vi "Initialize DAQ Channel.vi"(8 "error in (no error)":errorcluster, 10 "DAQmx Analog Channel":tag, 11 "DAQ AI in":refnum<class "DAQ AI.lvclass">) -> (0 "error out":errorcluster, 3 "DAQ AI out":refnum<class "DAQ AI.lvclass">)   [LabVIEW 2020, in "DAQ AI.lvlib" / "DAQ AI.lvclass"]
uses:
  DAQ AI.lvclass
  DAQ AI.lvclass/DAQ AI.ctl
  <vilib>/DAQmx/create/channels.llb/DAQmx Create Channel (AI-Voltage-Basic).vi
  <vilib>/DAQmx/configure/timing.llb/DAQmx Timing (Sample Clock).vi
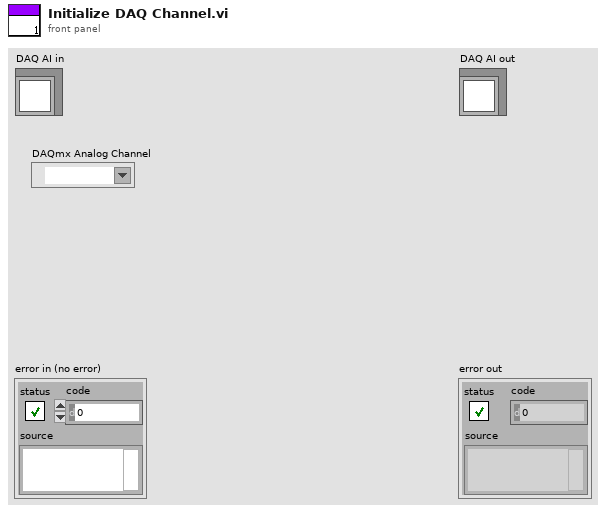
[diagram p1: front panel]
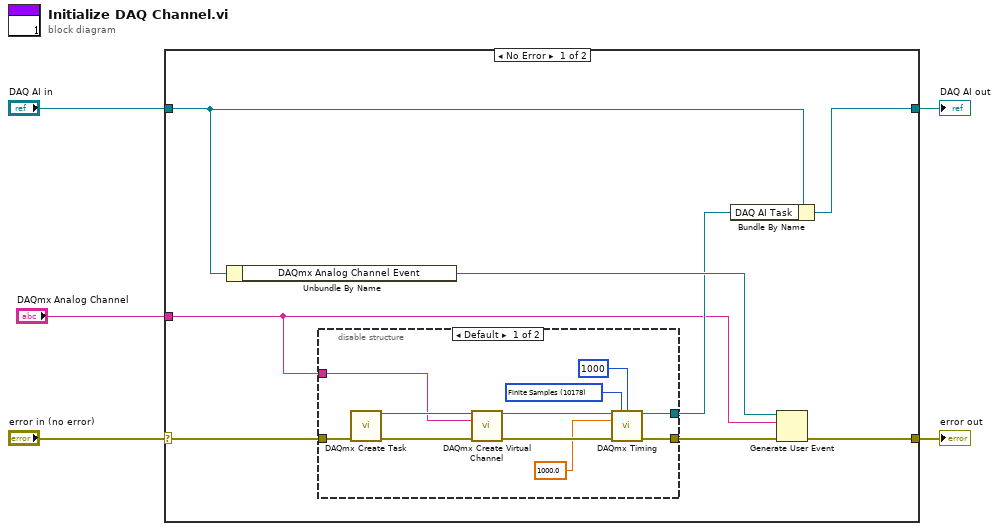
[diagram p0: block diagram]
diagram:
  n1 = case shown="No Error" "error in (no error)" {
    selector: "error in (no error)" -> [w12 w27]
    tunnel: [w9 w27] -> w4
    tunnel: [w13 w26] -> w2
    tunnel: "DAQ AI in" -> [w11 w26]
    tunnel: "DAQmx Analog Channel" -> [w6 _]
    frame No Error {
      n2 = Unbundle By Name(w11) -> ("DAQmx Analog Channel Event"=w10:refnum<user-event>)
      n3 = disable-structure shown="Default" {
        disable-tunnel: w12 -> [w22 w25]
        disable-tunnel: [w20 _] -> w8
        disable-tunnel: [w18 w25] -> w7
        disable-tunnel: w6 -> [w14 _]
        frame condition #0 (active) {
          w17 = 10178 items=["Finite Samples"=10178, "Continuous Samples"=10123, "Hardware Timed Single Point"=12522] ("sample mode")
          n4 = call <vilib>:"DAQmx Create Task.vi"("error in"=w22) -> ("task out"=w24:refnum<k21>, "error out"=w23:errorcluster)  [unwired: 13 in]
          n5 = call-poly <vilib>:"DAQmx Create Virtual Channel.vi"("task in"=w24, "physical channels"=w14, "error in"=w23) -> ("task out"=w21:refnum<k21>, "error out"=w19:errorcluster)  [unwired: 11 in]
          n6 = call-poly <vilib>:"DAQmx Timing.vi"("task/channels in"=w21, "sample mode"=w17, "samples per channel"=1000, "rate"=1000.0, "error in"=w19) -> ("task out"=w20:refnum<k21>, "error out"=w18:errorcluster)  [unwired: 9 in]
        }
        frame condition #1 {
        }
      }
      n7 = Bundle By Name(cluster=w11, "DAQ AI Task"=w8) -> (w13:refnum<class "DAQ AI.lvclass">)
      n8 = Generate User Event(user event=w10, event data cluster=w6, error in=w7) -> (error out=w9:errorcluster)  [unwired: 1 in, 1 out]
    }
    frame Error {
    }
  }
  "error out" <- w4
  "DAQ AI out" <- w2
